vi "空调初始化变量(子VI).vi"(8 "错误输入（无错误）":errorcluster) -> (0 "错误输出":errorcluster)   [LabVIEW 2016, in "环境动力监测库.lvlib" / "空调库.lvlib"]
uses:
  <vilib>/Utility/config.llb/NI_LVConfig.lvlib
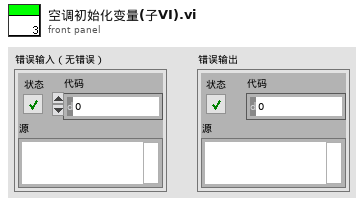
[diagram p1: front panel]
types:
  T1 = cluster{"监测项描述:输出":string, "连接方式":enum16{"串口", "TCP"}, "端口":string, "IP address:":string, "Port:":string, "站号":u64, "传感器型号":string, "波特率":u64, "data bits":u64, "停止位":u16, "奇偶校验":u16, "声光告警启用":bool}
  T2 = cluster{"baud rate (bps)":u32, "stop bits":u16, "parity":u16, "flow control":u16, "timeout":u32, "retries":i32}
  T3 = typedef "NI_LVConfig.lvlib/Config Data RefNum.ctl" = refnum<k1>
  T4 = cluster{"型号选择":enum16{"黑盾", "英维克", "仁科测控RS-KTC-N01"}, "MB session in":refnum<class "MB_Master.lvclass">, "英维克空调寄存器":u16[], "通讯状态":bool, "PORT":string, "IP":string, "Slave ID ":u8, "Serial Config":cluster{"baud rate (bps)":u32, "stop bits":u16, "parity":u16, "flow control":u16, "timeout":u32, "retries":i32}, "VISA Resource":refnum<visa-resource-name>, "MB通信方式选择":enum16{"串口", "TCP"}, "系统参数":cluster{"空调开启点":u16, "空调灵敏点":u16, "加热开启点":u16, "加热灵敏度":u16, "高温告警点":u16, "低温告警点":u16}}
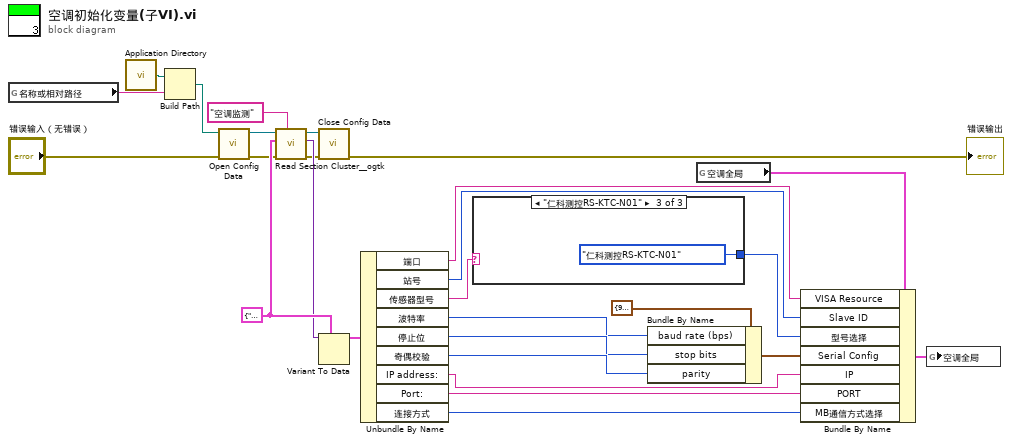
[diagram p0: block diagram]
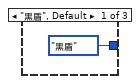
[diagram p2: hidden frame]
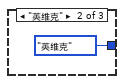
[diagram p3: hidden frame]
diagram:
  w27 = T1 {"监测项描述:输出"="", "连接方式"=enum."串口", "端口"="", "IP address:"="", "Port:"="", "站号"=19200, "传感器型号"="", "波特率"=19200, "data bits"=8, "停止位"=10, "奇偶校验"=0, "声光告警启用"=FALSE} ("输入簇")
  n1 = global read "内部交互全局变量.vi" "名称或相对路径"() -> (w1:string)
  n2 = call <vilib>:"Application Directory.vi"() -> ("Application Directory"=w5:path)
  n3 = Build Path(base path=w5, name or relative path=w1) -> (appended path=w4:path)
  n4 = call <vilib>:"Open Config Data.vi"("error in (no error)"="错误输入（无错误）", "configuration file path"=w4) -> ("error out"=w3:errorcluster, "refnum"=w2:T3)  [unwired: 7 in, 1 out]
  n5 = call <userlib>:"Read Section Cluster__ogtk.vi"("section (optional)"="空调监测", "error in (no error)"=w3, "Section Formatted Cluster Type"=w27, "refnum"=w2) -> ("error out"=w8:errorcluster, "Section Formatted Cluster"=w9:variant, "dup refnum"=w7:T3)  [unwired: 3 in, 2 out]
  n6 = call <vilib>:"Close Config Data.vi"("error in (no error)"=w8, "refnum"=w7) -> ("error out"=→"错误输出":errorcluster)  [unwired: 8 in, 1 out]
  n7 = Variant To Data(type=w27, Variant=w9) -> (data=w10:T1)  [unwired: 1 in, 1 out]
  n8 = Unbundle By Name(w10) -> ("端口"=w21:string, "站号"=w18:u64, "传感器型号"=w15:string, "波特率"=w12:u64, "停止位"=w13:u16, "奇偶校验"=w14:u16, "IP address:"=w23:string, "Port:"=w24:string, "连接方式"=w25:enum16{"串口", "TCP"})
  n9 = case shown="\"仁科测控RS-KTC-N01\"" w15 {
    tunnel: [enum16{"黑盾", "英维克", "仁科测控RS-KTC-N01"}."黑盾" ("型号选择") enum16{"黑盾", "英维克", "仁科测控RS-KTC-N01"}."英维克" ("型号选择") enum16{"黑盾", "英维克", "仁科测控RS-KTC-N01"}."仁科测控RS-KTC-N01" ("型号选择")] -> w20
    frame "黑盾", Default {
    }
    frame "英维克" {
    }
    frame "仁科测控RS-KTC-N01" {
    }
  }
  n10 = Bundle By Name(cluster=T2 {"baud rate (bps)"=9600, "stop bits"=10, "parity"=0, "flow control"=0, "timeout"=1000, "retries"=1} ("Serial Config"), "baud rate (bps)"=w12, "stop bits"=w13, "parity"=w14) -> (w22:T2)
  n11 = global read "断电保存全局变量.vi" "空调全局"() -> (w17:T4)
  n12 = Bundle By Name(cluster=w17, "VISA Resource"=w21, "Slave ID"=w18, "型号选择"=w20, "Serial Config"=w22, "IP"=w23, "PORT"=w24, "MB通信方式选择"=w25) -> (w19:T4)
  n13 = global write "断电保存全局变量.vi" "空调全局"(w19) -> ()
